vi "DSF.Shared.Configuration.Framework.Unique Name.Transfer.vi"(8 "error in (no error)":errorcluster, 10 "Transfer name in":string, 11 "Framework Configuration in":refnum<class "DSF.Shared.Configuration.Framework.lvclass">) -> (0 "error out":errorcluster, 1 "unique Transfer name?":bool, 2 "Transfer name out":string, 3 "Framework Configuration out":refnum<class "DSF.Shared.Configuration.Framework.lvclass">)   [LabVIEW 2016, in "DSF.Shared.lvlib" / "DSF.Shared.Configuration.Framework.lvclass"]
uses:
  DSF.Shared.Configuration.Framework.lvclass
  DSF.Shared.Configuration.Framework.lvclass/DSF.Shared.Configuration.Framework.ctl
  Configuration/DSF.Shared.Configuration.lvclass/DSF.Shared.Configuration.ctl
  Transfer/DSF.Shared.Configuration.Transfer.lvclass
  C:/Git/Sourcetree/DSF/Source/Shared/Classes/Configuration/DSF.Shared.Configuration.lvclass
  Configuration/DSF.Shared.Configuration.lvclass
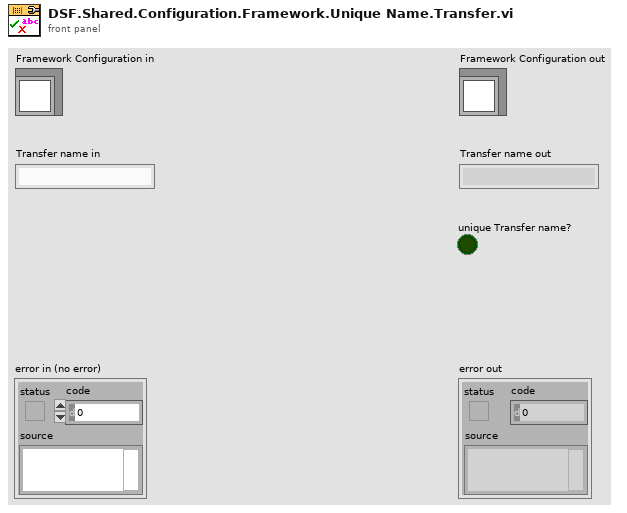
[diagram p1: front panel]
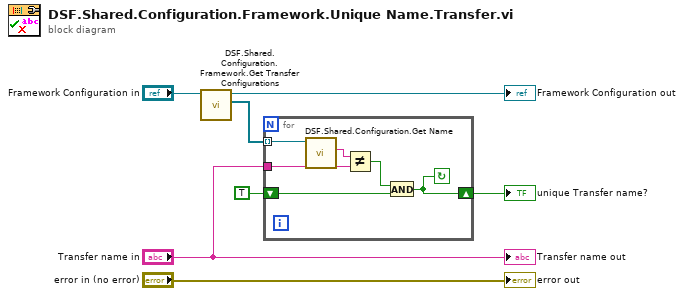
[diagram p0: block diagram]
diagram:
  n1 = call "DSF.Shared.Configuration.Framework.Get Transfer Configurations.vi"("Framework Configuration in"="Framework Configuration in") -> ("Transfer Configurations"=w6:refnum<class "DSF.Shared.Configuration.Transfer.lvclass">[], "Framework Configuration out"=→"Framework Configuration out":refnum<class "DSF.Shared.Configuration.Framework.lvclass">)  [unwired: 9 in]
  n2 = for {
    tunnel: w6 -> [w13] mode=indexing
    tunnel: "Transfer name in" -> [w11]
    shift-right: [w8] -> w4
    shift-left: TRUE -> [w10]
    stop <- w8 continue-if-true
    n3 = call "DSF.Shared.Configuration.Get Name.vi"("Configuration in"=w13) -> ("name"=w12:string)  [unwired: 9 in, 1 out]
    n4 = Not Equal?(x=w12, y=w11) -> (x != y?=w9:bool)
    n5 = And(x=w9, y=w10) -> (x .and. y?=w8:bool)
  }
  "unique Transfer name?" <- w4
  "error out" <- "error in (no error)"
  "Transfer name out" <- "Transfer name in"
